vi "Continuous Aq Daqmx.vi"() -> ()   [LabVIEW 2020]
uses:
  <vilib>/DAQmx/read.llb/DAQmx Read (Analog 1D Wfm NChan NSamp).vi
  <vilib>/DAQmx/miscellaneous.llb/DAQmx Fill In Error Info.vi
panel:
  in  "stop":bool
  out "Waveform Graph":waveform(dbl)[](graph)
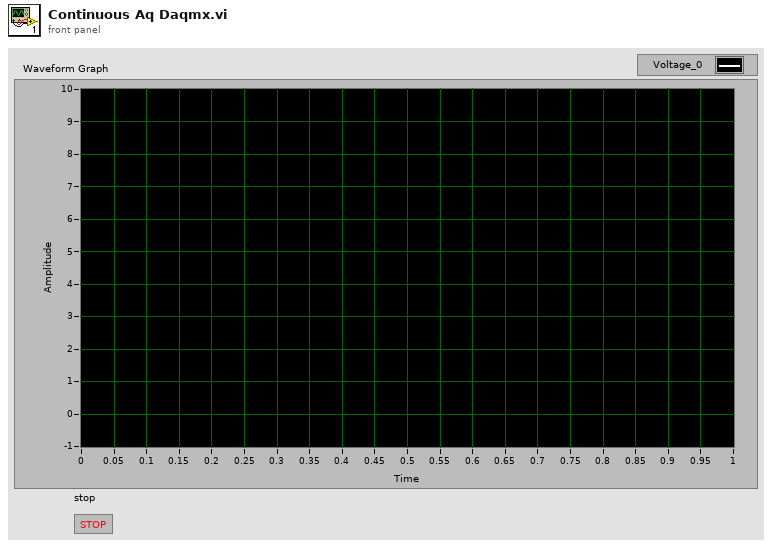
[diagram p1: front panel]
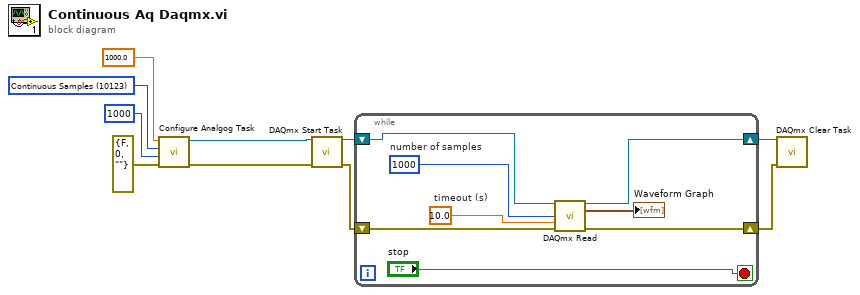
[diagram p0: block diagram]
diagram:
  w5 = 10123 items=["Finite Samples"=10178, "Continuous Samples"=10123, "Hardware Timed Single Point"=12522] ("sample mode")
  n1 = call "Configure Analgog Task.vi"("error in"=errorcluster {"status"=FALSE, "code"=0, "source"=""}, "number of samples"=1000, "sample mode"=w5, "rate"=1000.0) -> ("error out"=w8:errorcluster, "task out"=w2:refnum<k21>)  [unwired: 6 in]
  n2 = call <vilib>:"DAQmx Start Task.vi"("task/channels in"=w2, "error in"=w8) -> ("task out"=w1:refnum<k21>, "error out"=w3:errorcluster)  [unwired: 12 in]
  n3 = while {
    shift-right: [w15] -> w9
    shift-left: w1 -> [w14]
    shift-right: [w16] -> w10
    shift-left: w3 -> [w13]
    stop <- "stop" stop-if-true
    w17 = 10.0  # timeout (s)
    w18 = 1000  # number of samples
    n4 = call-poly <vilib>:"DAQmx Read.vi"("task/channels in"=w14, "number of samples per channel"=w18, "timeout"=w17, "error in"=w13) -> ("task out"=w15:refnum<k21>, "data"=→"Waveform Graph":waveform(dbl)[], "error out"=w16:errorcluster)  [unwired: 9 in]
  }
  n5 = call <vilib>:"DAQmx Clear Task.vi"("task in"=w9, "error in"=w10) -> ()  [unwired: 13 in, 1 out]
